vi "HTS_CALC_ACQUISITION_TIME.vi"(1 "Loader Settings":T1 {"Sample Volume (uL)" min=2.0 max=200.0 step=0.5; "Mixing Volume (uL)" min=5 max=100 step=5; "Mixing Speed (uL/s)" min=25 max=250 step=5; "Sample Flow Rate (uL/s)" min=0.5 max=3.0 step=0.5 format="%_2f"; "Mix#" min=0 max=5 step=1; "Wash Volume (uL)" min=200 max=800 step=20}) -> (0 "Numeric":u32)   [LabVIEW 2009]
uses:
  HTS_LOADER_SETTINGS.ctl
  HTS_INJECTION_MODE.ctl
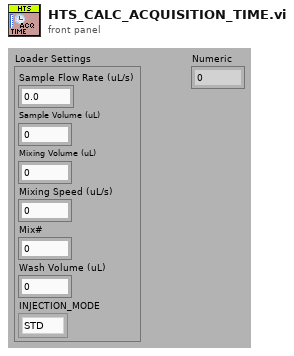
[diagram p1: front panel]
types:
  T1 = typedef "HTS_LOADER_SETTINGS.ctl" = cluster{"Sample Flow Rate (uL/s)":dbl, "Sample Volume (uL)":dbl, "Mixing Volume (uL)":i32, "Mixing Speed (uL/s)":i32, "Mix#":i32, "Wash Volume (uL)":i32, "INJECTION_MODE":T2}
  T2 = typedef "HTS_INJECTION_MODE.ctl" = enum16{"STD", "HT"}
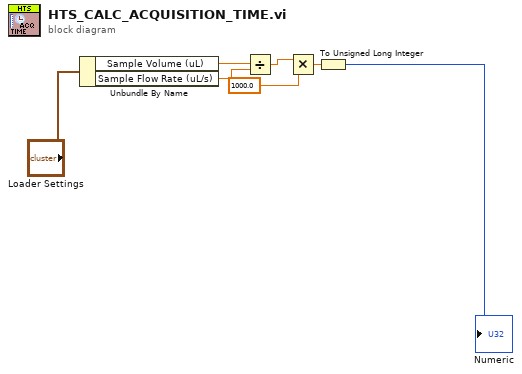
[diagram p0: block diagram]
diagram:
  n1 = Unbundle By Name("Loader Settings") -> ("Sample Volume (uL)"=w2:dbl, "Sample Flow Rate (uL/s)"=w3:dbl)
  n2 = Divide(x=w2, y=w3) -> (x/y=w4:dbl)
  n3 = Multiply(x=w4, y=1000.0) -> (x*y=w6:dbl)
  n4 = To Unsigned Long Integer(number=w6) -> (unsigned 32bit integer=→"Numeric":u32)
